vi "Read Header File and Populate String Array.vi"(0 "file path (dialog if empty)":path, 5 "error in (no error)":errorcluster) -> (14 "subarray":string[](array[string]), 19 "error out":errorcluster)   [LabVIEW 2015]
doc: "This vi reads a txt file containing the list of column names and returns them in an array"
uses:
  <vilib>/Utility/file.llb/Read From Spreadsheet File (string).vi
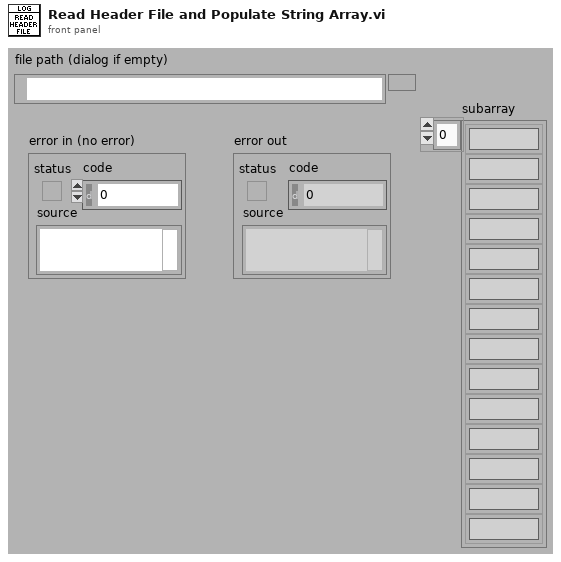
[diagram p1: front panel]
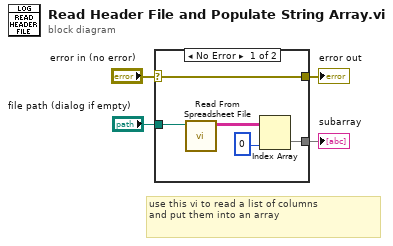
[diagram p0: block diagram]
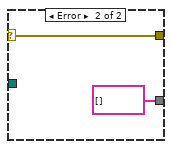
[diagram p2: hidden frame]
diagram:
  # "use this vi to read a list of columns\nand put them into an array"
  n1 = case shown="No Error" "error in (no error)" {
    selector: "error in (no error)" -> [w5 w11]
    tunnel: "file path (dialog if empty)" -> [w9 _]
    tunnel: [w7 string[] [] ("all rows")] -> w3
    tunnel: [w5 w11] -> w1
    frame No Error {
      n2 = call-poly <vilib>:"Read From Spreadsheet File.vi"("file path (dialog if empty)"=w9) -> ("all rows"=w8:string[][])  [unwired: 6 in, 4 out]
      n3 = Index Array(array=w8, index (col)=0 ("index (row)")) -> (element=w7:string[])  [unwired: 1 in]
    }
    frame Error {
    }
  }
  "subarray" <- w3
  "error out" <- w1
